vi "_readString.vi"(8 "error in (no error)":errorcluster, 11 "JSONParser in":refnum<class "tJSONParser.lvclass">) -> (0 "error out":errorcluster, 2 "String":string, 3 "JSONParser out":refnum<class "tJSONParser.lvclass">)   [LabVIEW 2013, in "JSON.lvlib" / "tJSONParser.lvclass"]
doc: "Reads and validates a string. Errors if EOF or EOL is ecountered before the closing double quote."
uses:
  tJSONParser.lvclass
  tJSONParser.lvclass/tJSONParser.ctl
  _error.ctl
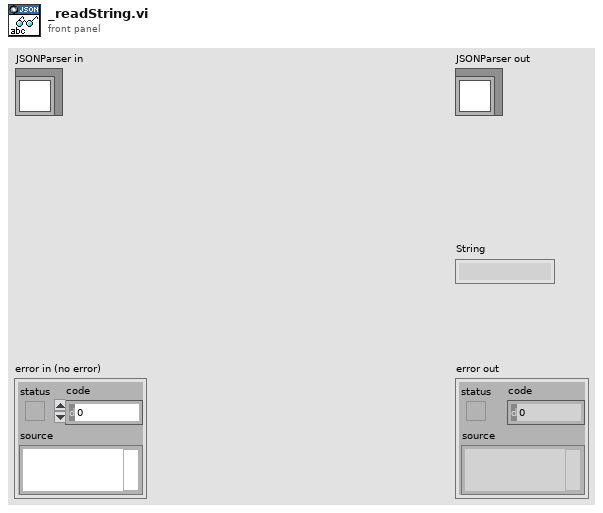
[diagram p1: front panel]
types:
  T1 = typedef "JSON.lvlib/tJSONParser.lvclass/_error.ctl" = enum16{"Missing Object Open", "Missing Pair Separator", "Missing Object End Or Separator", "Missing Pair String", "Unexpected Token", "Missing Array End Or Separator", "Invalid Escape Sequence", "Unexpected End Of File", "Invalid Unicode", "Unexpected End Of Line", "Invalid Numerical Constant"}
  T2 = typedef "JSON.lvlib/tJSONParser.lvclass/_tokenType.ctl" = enum16{"Object Begin", "Object End", "Array Begin", "Array End", "String Delimeter", "Forward Slash", "Number", "Boolean", "Null", "Object Or Array Separator", "Pair Separator", "End Of File", "Asterisk", "Backward Slash", "Other"}
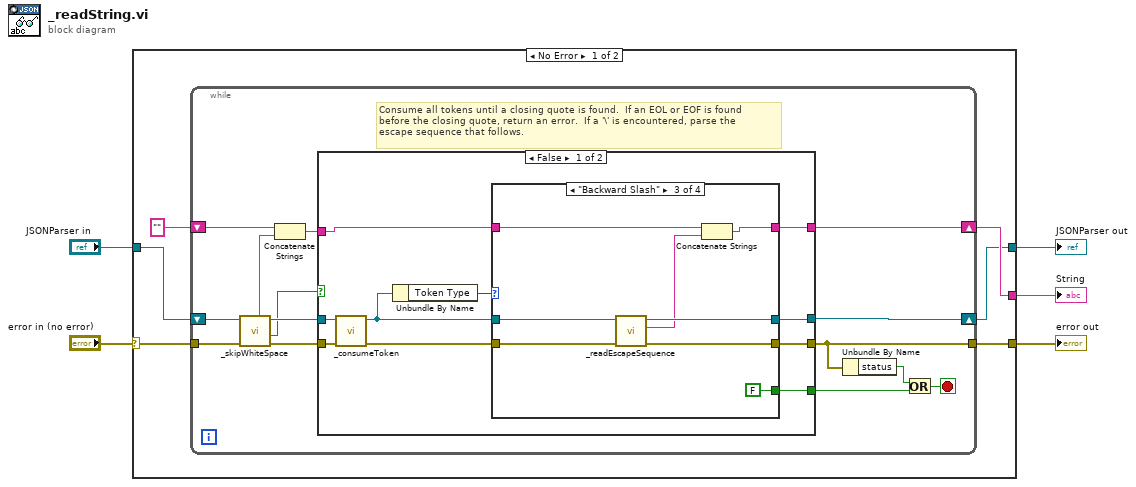
[diagram p0: block diagram]
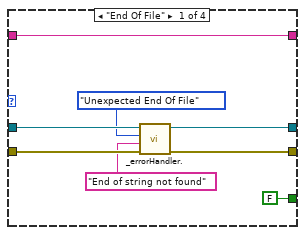
[diagram p2: hidden frame]
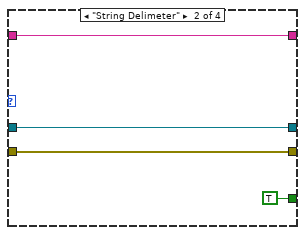
[diagram p3: hidden frame]
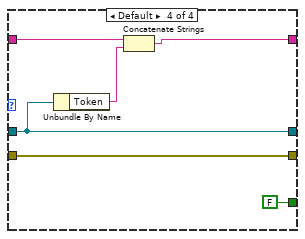
[diagram p4: hidden frame]
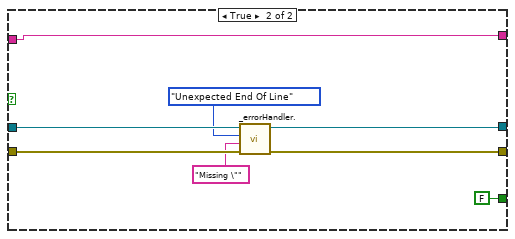
[diagram p5: hidden frame]
diagram:
  n1 = case shown="No Error" "error in (no error)" {
    selector: "error in (no error)" -> [w11 w71]
    tunnel: [w9 w71] -> w4
    tunnel: [w6 w70] -> w2
    tunnel: "JSONParser in" -> [w10 w70]
    tunnel: [w7 _] -> w1
    frame No Error {
      n2 = while {
        tunnel: w11 -> [w18]
        tunnel: [w24] -> w9
        shift-right: [w20] -> w7
        shift-left: "" -> [w16]
        shift-right: [w12] -> w6
        shift-left: w10 -> [w25]
        stop <- w22 stop-if-true
        # "Consume all tokens until a closing quote is found.  If an EOL or EOF is found\nbefore the closing quote, return an error.  If a '\\' is encountered, parse the\nescape sequence that follows."
        n3 = call "_skipWhiteSpace.vi"("error in (no error)"=w18, "JSON Parser In"=w25) -> ("error out"=w17:errorcluster, "EOL Found?"=w13:bool, "JSON Parser Out"=w19:refnum<class "tJSONParser.lvclass">, "Whitespace String"=w14:string)  [unwired: 5 in, 1 out]
        n4 = Concatenate Strings(w16, w14) -> (w15:string)
        n5 = case shown="False" w13 {
          tunnel: [w32 w66] -> w24
          tunnel: [w31 FALSE] -> w21
          tunnel: [w30 w68] -> w20
          tunnel: w19 -> [w29 w65]
          tunnel: w17 -> [w28 w67]
          tunnel: w15 -> [w27 w68]
          tunnel: [w26 w62] -> w12
          frame False {
            n6 = call "_consumeToken.vi"("error in (no error)"=w28, "JSON Parser In"=w29) -> ("error out"=w33:errorcluster, "JSON Parser Out"=w34:refnum<class "tJSONParser.lvclass">)  [unwired: 8 in]
            n7 = Unbundle By Name(w34) -> ("Token Type"=w35:T2)
            n8 = case shown="\"Backward Slash\"" w35 {
              tunnel: w34 -> [w40 w46 w48 w58]
              tunnel: w33 -> [w43 w47 w53 w61]
              tunnel: [w42 w47 w52 w61] -> w32
              tunnel: [w41 w46 w54 w58] -> w26
              tunnel: [FALSE TRUE FALSE FALSE] -> w31
              tunnel: w27 -> [w36 w44 w51 w59]
              tunnel: [w36 w44 w50 w56] -> w30
              frame "End Of File" {
                n9 = call "_errorHandler..vi"("error in (no error)"=w43, "Additional Text"="End of string not found", "Error Type"=_error."Unexpected End Of File", "JSON Parser In"=w40) -> ("error out"=w42:errorcluster, "JSON Parser Out"=w41:refnum<class "tJSONParser.lvclass">)  [unwired: 6 in]
              }
              frame "String Delimeter" {
              }
              frame "Backward Slash" {
                n10 = call "_readEscapeSequence.vi"("error in (no error)"=w53, "tJSONParser in"=w48) -> ("error out"=w52:errorcluster, "String Out"=w49:string, "tJSONParser out"=w54:refnum<class "tJSONParser.lvclass">)  [unwired: 7 in]
                n11 = Concatenate Strings(w51, w49) -> (w50:string)
              }
              frame Default {
                n12 = Unbundle By Name(w58) -> ("Token"=w57:string)
                n13 = Concatenate Strings(w59, w57) -> (w56:string)
              }
            }
          }
          frame True {
            n14 = call "_errorHandler..vi"("error in (no error)"=w67, "Additional Text"="Missing \"", "Error Type"=_error."Unexpected End Of Line", "JSON Parser In"=w65) -> ("error out"=w66:errorcluster, "JSON Parser Out"=w62:refnum<class "tJSONParser.lvclass">)  [unwired: 6 in]
          }
        }
        n15 = Unbundle By Name(w24) -> ("status"=w23:bool)
        n16 = Or(x=w23, y=w21) -> (x .or. y?=w22:bool)
      }
    }
    frame Error {
    }
  }
  "error out" <- w4
  "JSONParser out" <- w2
  "String" <- w1
